vi "Eth Status Write Inputs.vi"(7 "Status Reference":T1, 8 "error in (no error)":errorcluster, 9 "Write Enable":bool[](array[boolean]), 10 "Start":bool[](array[boolean]), 11 "Lenght":i32) -> (0 "error out":errorcluster, 5 "Status Reference out":T1)   [LabVIEW 2021, in "Eth Status.lvlib"]
uses:
  Eth Status.lvlib
  Ctl/Status.ctl
  MB_TCP2/MB_TCP_State.ctl
  MB_TCP2/MB_TCP.lvclass
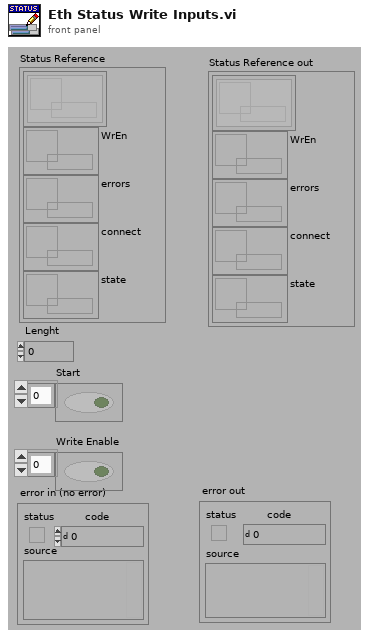
[diagram p1: front panel]
types:
  T1 = typedef "Eth Status.lvlib/Status.ctl" = cluster{"Set_states":refnum<queue>[], "WrEn":refnum<data-value>, "errors":refnum<data-value>, "connect":refnum<data-value>, "state":refnum<data-value>}
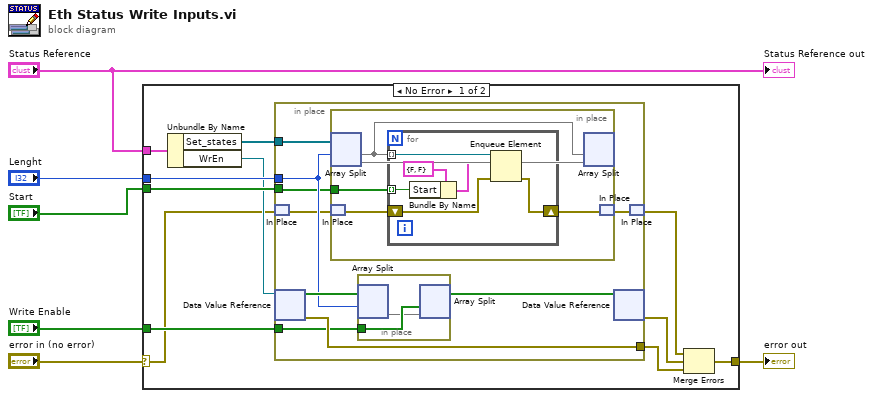
[diagram p0: block diagram]
diagram:
  n1 = case shown="No Error" "error in (no error)" {
    selector: "error in (no error)" -> [w8 w40]
    tunnel: [w15 w40] -> w5
    tunnel: "Lenght" -> [w17 _]
    tunnel: "Status Reference" -> [w16 _]
    tunnel: "Start" -> [w14 _]
    tunnel: "Write Enable" -> [w13 _]
    frame No Error {
      n2 = Unbundle By Name(w16) -> ("Set_states"=w9:refnum<queue>[], "WrEn"=w10:refnum<data-value>)
      n3 = in-place {
        in-place-border: w17 -> [w21]
        in-place-border: w14 -> [w20]
        in-place-border: w13 -> [w24]
        in-place-border: [w26] -> w11
        in-place-border: w9 -> [w22]
        n4 = in-place-match #1(w8) -> (w19:errorcluster)
        n5 = in-place-dvr #2(w10) -> (w25:bool[], w26:errorcluster)
        n6 = in-place {
          in-place-border: w20 -> [w29]
          n7 = in-place-split #3(w22, w21) -> (w31:refnum<queue>[], w30:refnum<queue>[])
          n8 = in-place-match #4(w19) -> (w28:errorcluster)
          n9 = for {
            tunnel: w31 -> [w37] mode=indexing
            shift-right: [w35] -> w27
            shift-left: w28 -> [w36]
            tunnel: w29 -> [w32] mode=indexing
            n10 = Bundle By Name(cluster=cluster{"Start":bool, "Stop":bool} {"Start"=FALSE, "Stop"=FALSE} ("element"), "Start"=w32) -> (w33:cluster{"Start":bool, "Stop":bool})
            n11 = Enqueue Element(queue=w37, element=w33, error in (no error)=w36) -> (error out=w35:errorcluster)  [unwired: 1 in, 2 out]
          }
          n12 = in-place-split #3(w31, w30) -> ()  [unwired: 2 out]
          n13 = in-place-match #4(w27) -> (w18:errorcluster)
        }
        n14 = in-place {
          in-place-border: w24 -> [w39]
          n15 = in-place-split #5(w25, w21) -> (w38:bool[])  [unwired: 1 out]
          n16 = in-place-split #5(w39, w38) -> (w23:bool[])  [unwired: 1 out]
        }
        n17 = in-place-dvr #2(w23) -> (w12:errorcluster)  [unwired: 1 out]
        n18 = in-place-match #1(w18) -> (w7:errorcluster)
      }
      n19 = Merge Errors(w7, w12, w11) -> (w15:errorcluster)
    }
    frame Error {
    }
  }
  "error out" <- w5
  "Status Reference out" <- "Status Reference"
